vi "Test MC Heartbeat Message.vi"() -> ()   [LabVIEW 2015]
uses:
  Global Data.vi
panel:
  in  "Requested Torque (Nm)":dbl format="%#_13g"
  in  "HeartBeat/\nCommand message":bool
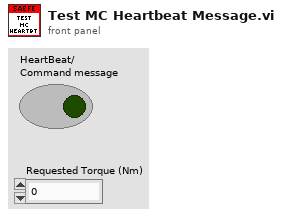
[diagram p1: front panel]
types:
  T1 = typedef "CAN Message Queue.ctl" = refnum<k33>
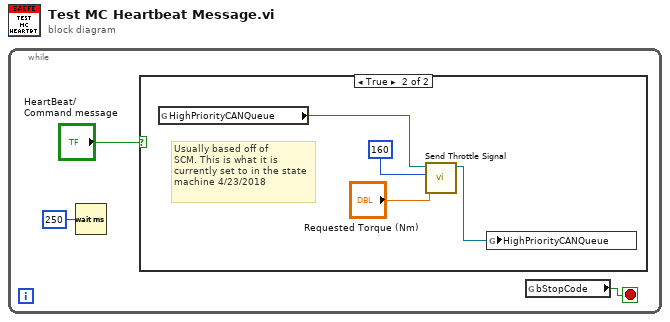
[diagram p0: block diagram]
diagram:
  n1 = while {
    stop <- w3 stop-if-true
    n2 = Wait (ms)(milliseconds to wait=u32 250) -> ()  [unwired: 1 out]
    n3 = case shown="True" "HeartBeat/\nCommand message" {
      frame False {
      }
      frame True {
        # "Usually based off of\nSCM. This is what it is\ncurrently set to in the state\nmachine 4/23/2018"
        n4 = global read "Global Data.vi" "HighPriorityCANQueue"() -> (w6:T1)
        n5 = call "Send Throttle Signal.vi"("Requested Torque (Nm)"="Requested Torque (Nm)", "CAN Offset"=u32 160, "CANTXQueueIn"=w6) -> ("CANTXQueueOut"=w7:T1)  [unwired: 8 in]
        n6 = global write "Global Data.vi" "HighPriorityCANQueue"(w7) -> ()
      }
    }
    n7 = global read "Global Data.vi" "bStopCode"() -> (w3:bool)
  }
